vi "fpga_status.vi"(8 "error in (no error)":errorcluster, 11 "5785_3.2GHz_one channel in":refnum<class "5785_3.2GHz_one channel.lvclass">) -> (0 "error out":errorcluster, 2 "pulse TX status":T1, 3 "5785_3.2GHz_one channel out":refnum<class "5785_3.2GHz_one channel.lvclass">)   [LabVIEW 2021, in "5785_3.2GHz_one channel.lvclass"]
uses:
  5785_3.2GHz_one channel.lvclass
  5785_3.2GHz_one channel.lvclass/5785_3.2GHz_one channel.ctl
  <vilib>/Utility/error.llb/Error Cluster From Error Code.vi
  <vilib>/rvi/errors/niLvFpgaAdjustHostInterfaceError.vi
  <vilib>/rvi/interface/nirviReadWriteControl/nirviReadWriteControl.xnode
  NiFpgaLv.dll
  <vilib>/rvi/interface/Simulation/niFpgaSimulationCallBeginRW.vi
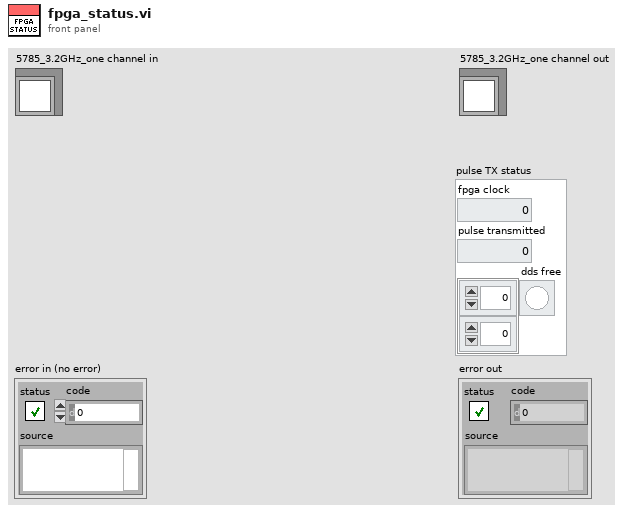
[diagram p1: front panel]
types:
  T1 = cluster{"fpga clock":dbl, "pulse transmitted":u32, "dds free":bool[][]}
  T2 = cluster{"fpga clock":u64, "pulse transmitted":u32, "dds free":bool[][]}
  T3 = cluster{"fpga clock":u64, "pulse transmitted":u32, "dds free":bool[]}
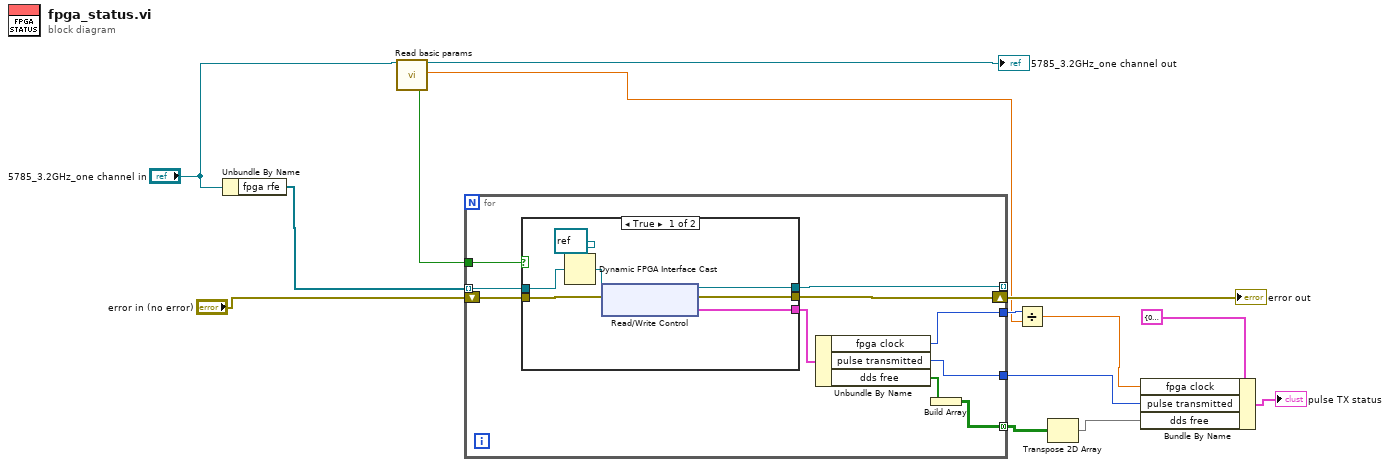
[diagram p0: block diagram]
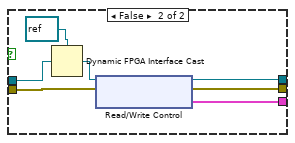
[diagram p2: hidden frame]
diagram:
  n1 = Unbundle By Name("5785_3.2GHz_one channel in") -> ("fpga rfe"=w2:refnum<k20>[])
  n2 = call-dynamic "Read basic params.vi"("device_type in"="5785_3.2GHz_one channel in") -> ("use arb files"=w1:bool, "device_type out"=→"5785_3.2GHz_one channel out":refnum<class "5785_3.2GHz_one channel.lvclass">, "Fs  FPGA"=w3:dbl)  [unwired: 12 in, 4 out]
  n3 = for {
    tunnel: w2 -> [w16] mode=indexing
    shift-right: [w23] -> w11
    shift-left: "error in (no error)" -> [w24]
    tunnel: [w22] -> _ mode=indexing
    tunnel: [w21] -> w13 mode=concatenating
    tunnel: [w18] -> w10
    tunnel: [w19] -> w14
    tunnel: w1 -> [w15]
    n4 = case shown="True" w15 {
      tunnel: w24 -> [w31 w38]
      tunnel: [w30 w37] -> w23
      tunnel: [w29 w36] -> w22
      tunnel: [w28 w35] -> w20
      tunnel: w16 -> [w26 w33]
      frame True {
        n5 = Dynamic FPGA Interface Cast(Session In=refnum<k20> refnum ("FPGA VI Reference Out"), Type=w26) -> (Session Out=w25:refnum<k20>)
        n6 = xnode "Read/Write Control"("FPGA VI Reference In"=w25, "error in"=w31) -> ("FPGA VI Reference Out"=w29:refnum<k20>, "error out"=w30:errorcluster, "pulse TX status"=w28:T3)
      }
      frame False {
        n7 = Dynamic FPGA Interface Cast(Session In=refnum<k20> refnum ("FPGA VI Reference Out"), Type=w33) -> (Session Out=w32:refnum<k20>)
        n8 = xnode "Read/Write Control"("FPGA VI Reference In"=w32, "error in"=w38) -> ("FPGA VI Reference Out"=w36:refnum<k20>, "error out"=w37:errorcluster, "pulse TX status"=w35:T3)
      }
    }
    n9 = Unbundle By Name(w20) -> ("fpga clock"=w19:u64, "pulse transmitted"=w18:u32, "dds free"=w17:bool[])
    n10 = Build Array(w17) -> (w21:bool[][])
  }
  "error out" <- w11
  n11 = Divide(x=w14, y=w3) -> (x/y=w9:dbl)
  n12 = Transpose 2D Array(2D array=w13) -> (transposed array=w6:bool[][])
  n13 = Bundle By Name(cluster=T2 {"fpga clock"=0, "pulse transmitted"=0, "dds free"=[[FALSE, FALSE, FALSE, FALSE, FALSE, FALSE, FALSE, FALSE, FALSE, FALSE, FALSE, FALSE, FALSE, FALSE, FALSE, FALSE]]} ("pulse TX status"), "fpga clock"=w9, "pulse transmitted"=w10, "dds free"=w6) -> (→"pulse TX status":T2)
